vi "Stop Logger.vi"(8 "error in (no error)":errorcluster, 11 "MsgQ in":refnum<class "MessageQ.lvclass">) -> (0 "error out":errorcluster, 3 "MsgQ":refnum<class "MessageQ.lvclass">)   [LabVIEW 2020, in "VolatusData.lvlib"]
uses:
  VolatusData.lvlib
  Volatus/MessageQ/MessageQ.lvclass
  Volatus/MessageQ/MessageQ.lvclass/MessageQ.ctl
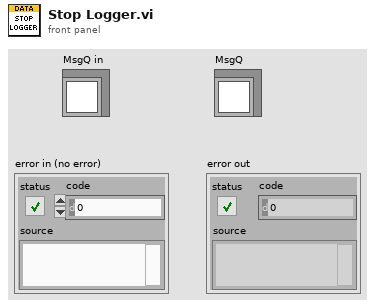
[diagram p1: front panel]
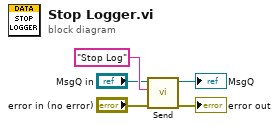
[diagram p0: block diagram]
diagram:
  n1 = call "Send.vi"("error in (no error)"="error in (no error)", "ID"="Stop Log", "MessageQ in"="MsgQ in") -> ("error out"=→"error out":errorcluster, "MessageQ out"=→"MsgQ":refnum<class "MessageQ.lvclass">)  [unwired: 7 in]
